vi "Log Write.vi"(0 "Error In":errorcluster, 1 "Write Header":bool, 5 "Log Handle In":T1, 7 "Trajectory In":refnum<data-value>, 9 "State Estimate In":refnum<data-value>, 11 "Measurement In":refnum<data-value>, 12 "Controller Data In":refnum<data-value>, 13 "Balance In":refnum<data-value>) -> (3 "Logged Events":string[](array[string]), 4 "Error Out":errorcluster, 6 "Log Handle Out":T1, 8 "Trajectory Out":refnum<data-value>, 10 "State Estimate Out":refnum<data-value>, 14 "Controller Data Out":refnum<data-value>, 15 "Measurement Out":refnum<data-value>)   [LabVIEW 2021]
uses:
  State Estimator/Measurements.ctl
  IMU/IMU Data.ctl
  Steering Motor Encoder/Steering Motor Encoder Data.ctl
  GNSS/GNSS Data.ctl
  State Estimator/State Estimate.ctl
  Log Handle.ctl
  Controller Data.ctl
  Drive Motor/Drive Motor Data.ctl
  Steering Motor/Steering Motor Data.ctl
  Trajectory Control/Trajectory_Control.ctl
panel:
  out "velocity":dbl
  out "GNSS Data.Speed (m/s)":dbl
  out "rollReference":dbl
  out "Balance Out":refnum<data-value>
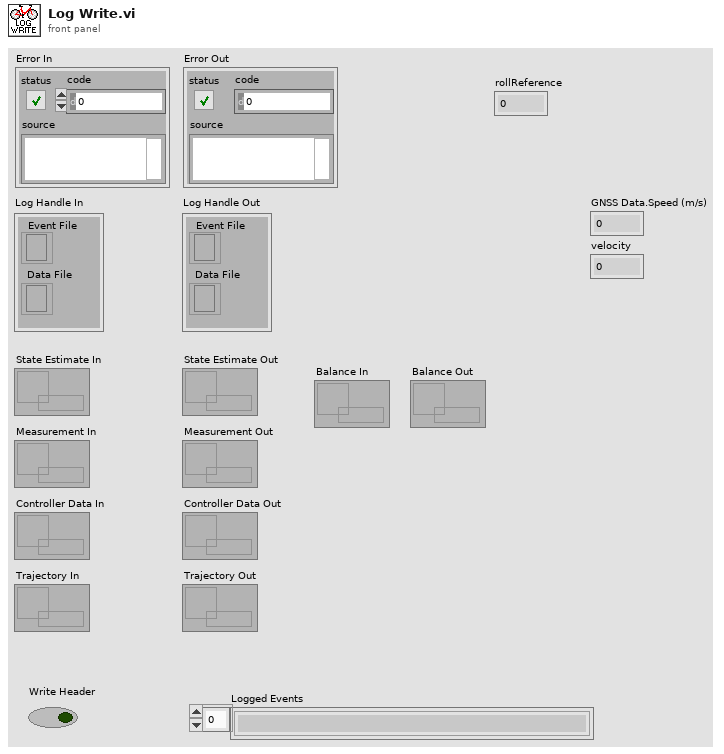
[diagram p1: front panel]
types:
  T1 = typedef "Log Handle.ctl" = cluster{"Data File":refnum<file>, "Event File":refnum<file>}
  T2 = typedef "Controller Data.ctl" = cluster{"Drive Motor Data":T3, "Steering Motor Data":T4}
  T3 = typedef "Drive Motor Data.ctl" = cluster{"Angular Speed (rad/s)":dbl, "Input Current (A)":dbl, "Motor Current (A)":dbl, "MOSFET Temperature (deg C)":dbl, "Reference Speed (rad/s)":dbl, "PI Current (A)":dbl, "Ki":dbl, "Kp":dbl}
  T4 = typedef "Steering Motor Data.ctl" = cluster{"PWM":dbl, "Steering Angle Rate (rad/s)":dbl, "input balancing":dbl}
  T5 = typedef "Trajectory_Control.ctl" = cluster{"Rollref":dbl, "Closestpoint":dbl, "Error1":dbl, "Error2":dbl, "Dpsiref_cont":dbl, "Lateral_cont":dbl, "Heading_cont":dbl, "Reset_traj":dbl, "Iteration":dbl, "E1 limit":u32, "E2 limit":u32}
  T6 = typedef "State Estimate.ctl" = cluster{"X (m)":dbl, "Y (m)":dbl, "Psi (rad)":dbl, "Roll (rad)":dbl, "Roll Rate (rad/s)":dbl, "delta":dbl, "velocity":dbl, "Iterations":dbl}
  T7 = cluster{"Steering Angle Rate":dbl, "rollReference":dbl, "roll":dbl, "rollRate":dbl, "Kp":dbl, "Kd":dbl, "steering_flag":i32}
  T8 = typedef "Measurements.ctl" = cluster{"IMU Data":T9, "Steering Motor Encoder Data":T10, "GNSS Data":T11}
  T9 = typedef "IMU Data.ctl" = cluster{"Gyroscope":cluster{"X (rad/s)":dbl, "Y (rad/s)":dbl, "Z (rad/s)":dbl}, "Accelerometer":cluster{"X (m/s^2)":dbl, "Y (m/s^2)":dbl, "Z (m/s^2)":dbl}, "Flag IMU":dbl}
  T10 = typedef "Steering Motor Encoder Data.ctl" = cluster{"Encoder Position (counts)":i32, "Steering Angle (rad)":dbl, "Steering Encoder Iteration":dbl}
  T11 = typedef "GNSS Data.ctl" = cluster{"Latitude (rad)":dbl, "Longitude (rad)":dbl, "Altitude (m)":dbl, "Speed (m/s)":dbl, "Heading (rad)":dbl, "Fix Quality":i32, "Number of Satellites":i32, "Latitude (deg)":dbl, "Longitude (deg)":dbl, "Flag GNSS":dbl}
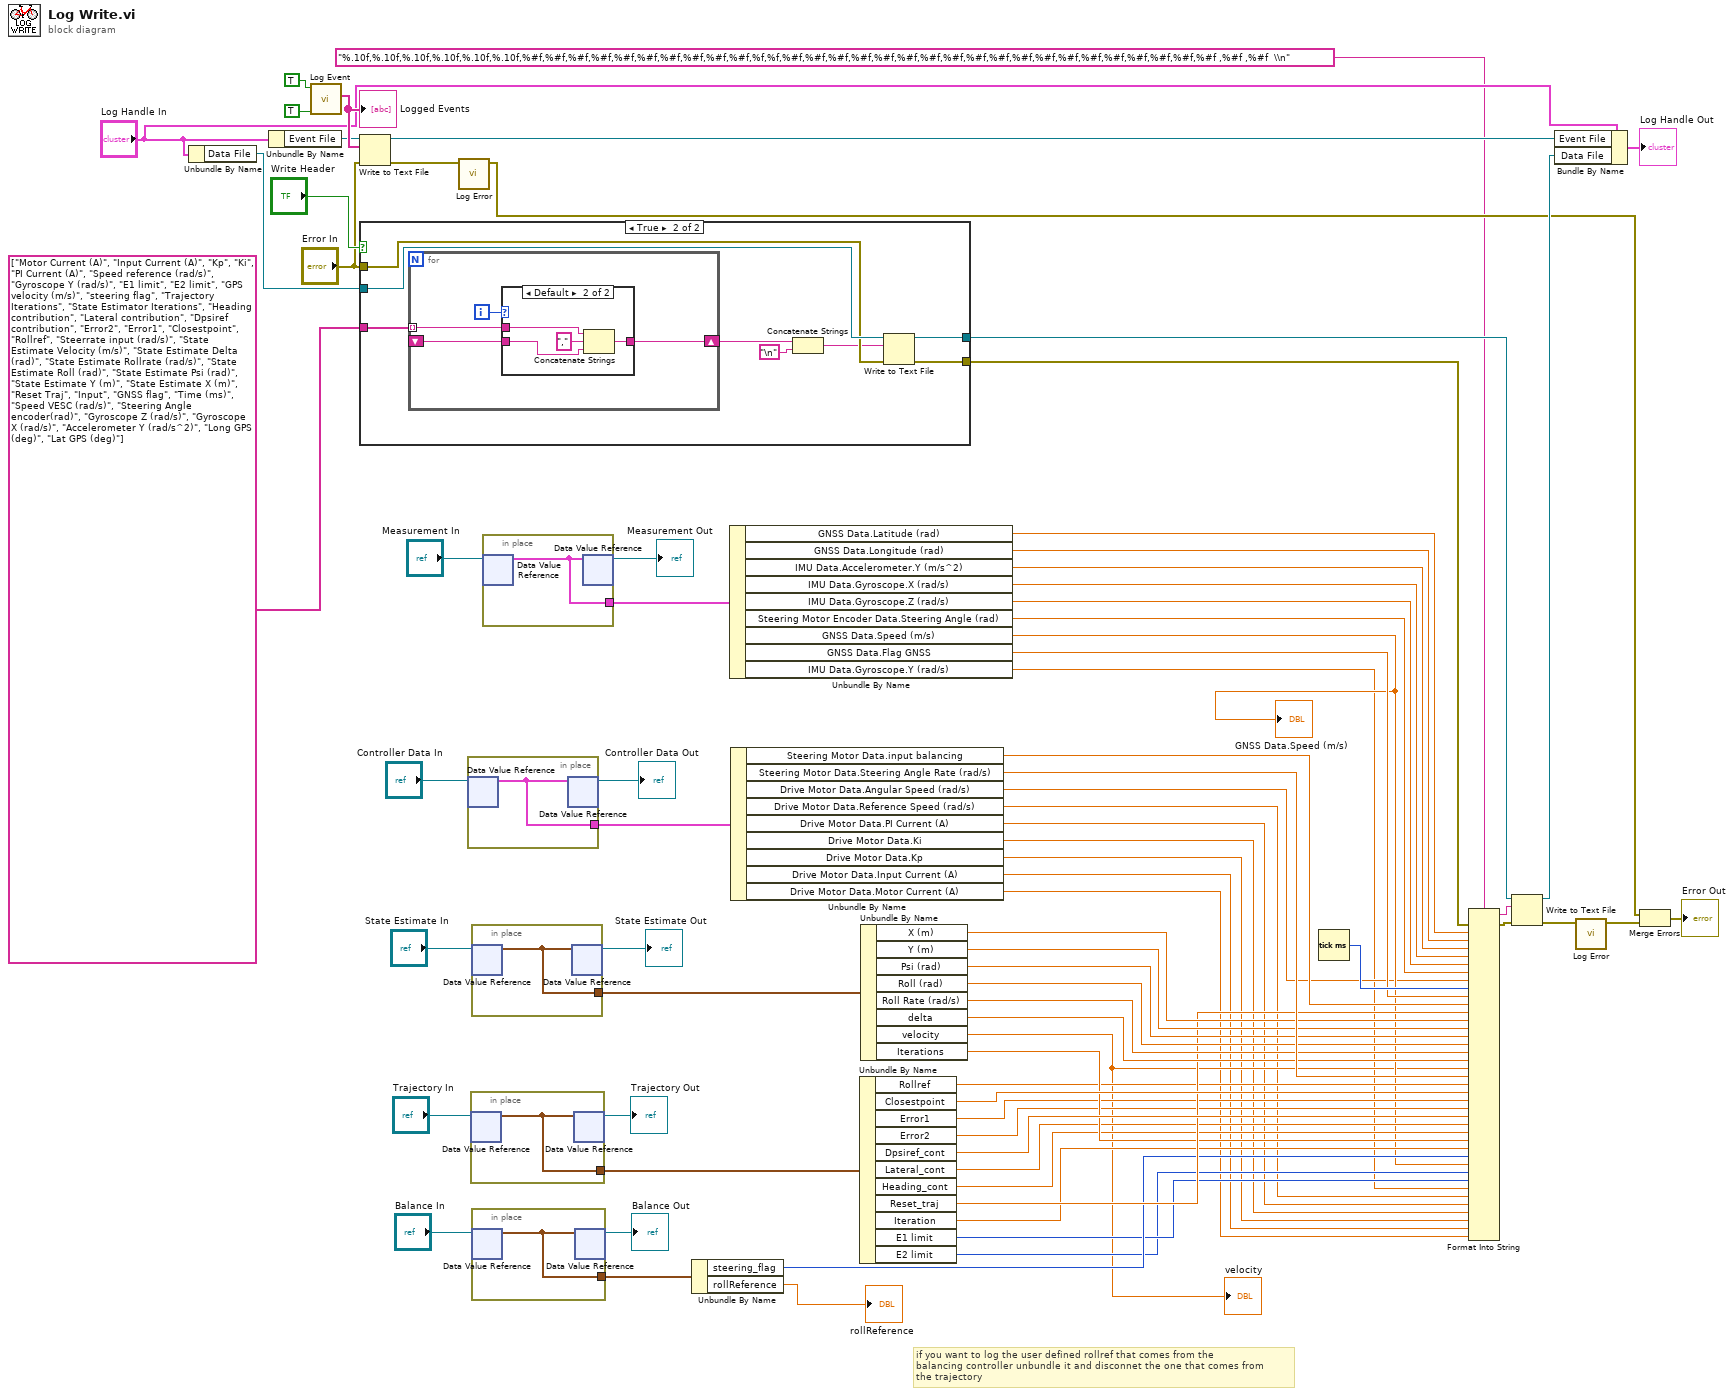
[diagram p0: block diagram]
diagram:
  # "if you want to log the user defined rollref that comes from the \nbalancing controller unbundle it and disconnet the one that comes from \nthe trajectory"
  n1 = Unbundle By Name("Log Handle In") -> ("Data File"=w76:refnum<file>)
  n2 = Unbundle By Name("Log Handle In") -> ("Event File"=w68:refnum<file>)
  n3 = call "Log Event.vi"("Clear Log"=TRUE, "Read"=TRUE) -> ("All Events"=w70:string[])  [unwired: 9 in]
  "Logged Events" <- w70
  n4 = Write to Text File(file (use dialog)=w68, text=w70, error in="Error In") -> (refnum out=w65:refnum<file>, error out=w64:errorcluster)  [unwired: 1 in, 1 out]
  n5 = case shown="True" "Write Header" {
    tunnel: string[] ["Motor Current (A)", "Input Current (A)", "Kp", "Ki", "PI Current (A)", "Speed reference (rad/s)", "Gyroscope Y (rad/s)", "E1 limit", "E2 limit", "GPS velocity (m/s)", "steering flag", "Trajectory Iterations", "State Estimator Iterations", "Heading contribution", "Lateral contribution", "Dpsiref contribution", "Error2", "Error1", "Closestpoint", "Rollref", "Steerrate input (rad/s)", "State Estimate Velocity (m/s)", "State Estimate Delta (rad)", "State Estimate Rollrate (rad/s)", "State Estimate Roll (rad)", "State Estimate Psi (rad)", "State Estimate Y (m)", "State Estimate X (m)", "Reset Traj", "Input", "GNSS flag", "Time (ms)", "Speed VESC (rad/s)", "Steering Angle encoder(rad)", "Gyroscope Z (rad/s)", "Gyroscope X (rad/s)", "Accelerometer Y (rad/s^2)", "Long GPS (deg)", "Lat GPS (deg)"] ("channel name(s) in (Untitled)") -> [_ w87]
    tunnel: w76 -> [w79 w86]
    tunnel: "Error In" -> [w78 w85]
    tunnel: [w79 w84] -> w74
    tunnel: [w78 w83] -> w73
    frame False {
    }
    frame True {
      n6 = for {
        tunnel: w87 -> [w91] mode=indexing
        shift-right: [w89] -> w82
        shift-left: _ -> [w88]
        i -> [w90]
        n7 = case shown="Default" w90 {
          tunnel: w91 -> [w92 w96]
          tunnel: [w92 w95] -> w89
          tunnel: w88 -> [_ w94]
          frame 0 {
          }
          frame Default {
            n8 = Concatenate Strings(w96, "," ("string"), w94) -> (w95:string)
          }
        }
      }
      n9 = Concatenate Strings(w82, "\n") -> (w81:string)
      n10 = Write to Text File(file (use dialog)=w86, text=w81, error in=w85) -> (refnum out=w84:refnum<file>, error out=w83:errorcluster)  [unwired: 1 in, 1 out]
    }
  }
  n11 = call "Log Error.vi"("Error In"=w64) -> ("Error Out"=w62:errorcluster)  [unwired: 10 in]
  n12 = in-place {
    in-place-border: [w97] -> w43
    n13 = in-place-dvr #1("Controller Data In") -> (w97:T2)  [unwired: 1 out]
    n14 = in-place-dvr #1(w97) -> (→"Controller Data Out":refnum<data-value>)  [unwired: 1 out]
  }
  n15 = in-place {
    in-place-border: [w98] -> w31
    n16 = in-place-dvr #2("Trajectory In") -> (w98:T5)  [unwired: 1 out]
    n17 = in-place-dvr #2(w98) -> (→"Trajectory Out":refnum<data-value>)  [unwired: 1 out]
  }
  n18 = in-place {
    in-place-border: [w99] -> w54
    n19 = in-place-dvr #3("State Estimate In") -> (w99:T6)  [unwired: 1 out]
    n20 = in-place-dvr #3(w99) -> (→"State Estimate Out":refnum<data-value>)  [unwired: 1 out]
  }
  n21 = in-place {
    in-place-border: [w100] -> w17
    n22 = in-place-dvr #4("Balance In") -> (w100:T7)  [unwired: 1 out]
    n23 = in-place-dvr #4(w100) -> (→"Balance Out":refnum<data-value>)  [unwired: 1 out]
  }
  n24 = in-place {
    in-place-border: [w101] -> w55
    n25 = in-place-dvr #5("Measurement In") -> (w101:T8)  [unwired: 1 out]
    n26 = in-place-dvr #5(w101) -> (→"Measurement Out":refnum<data-value>)  [unwired: 1 out]
  }
  n27 = Unbundle By Name(w17) -> ("steering_flag"=w16:i32, "rollReference"=→"rollReference":dbl)
  n28 = Unbundle By Name(w55) -> ("GNSS Data.Latitude (rad)"=w34:dbl, "GNSS Data.Longitude (rad)"=w53:dbl, "IMU Data.Accelerometer.Y (m/s^2)"=w52:dbl, "IMU Data.Gyroscope.X (rad/s)"=w51:dbl, "IMU Data.Gyroscope.Z (rad/s)"=w50:dbl, "Steering Motor Encoder Data.Steering Angle (rad)"=w49:dbl, "GNSS Data.Speed (m/s)"=w11:dbl, "GNSS Data.Flag GNSS"=w29:dbl, "IMU Data.Gyroscope.Y (rad/s)"=w8:dbl)
  "GNSS Data.Speed (m/s)" <- w11
  n29 = Unbundle By Name(w43) -> ("Steering Motor Data.input balancing"=w26:dbl, "Steering Motor Data.Steering Angle Rate (rad/s)"=w42:dbl, "Drive Motor Data.Angular Speed (rad/s)"=w10:dbl, "Drive Motor Data.Reference Speed (rad/s)"=w7:dbl, "Drive Motor Data.PI Current (A)"=w6:dbl, "Drive Motor Data.Ki"=w5:dbl, "Drive Motor Data.Kp"=w4:dbl, "Drive Motor Data.Input Current (A)"=w2:dbl, "Drive Motor Data.Motor Current (A)"=w1:dbl)
  n30 = Unbundle By Name(w31) -> ("Rollref"=w14:dbl, "Closestpoint"=w30:dbl, "Error1"=w21:dbl, "Error2"=w20:dbl, "Dpsiref_cont"=w28:dbl, "Lateral_cont"=w23:dbl, "Heading_cont"=w22:dbl, "Reset_traj"=w27:dbl, "Iteration"=w24:dbl, "E1 limit"=w13:u32, "E2 limit"=w12:u32)
  n31 = Unbundle By Name(w54) -> ("X (m)"=w40:dbl, "Y (m)"=w39:dbl, "Psi (rad)"=w38:dbl, "Roll (rad)"=w37:dbl, "Roll Rate (rad/s)"=w36:dbl, "delta"=w35:dbl, "velocity"=w9:dbl, "Iterations"=w25:dbl)
  "velocity" <- w9
  n32 = Tick Count (ms)() -> (millisecond timer value=w41:u32)
  n33 = Format Into String(format string="%.10f,%.10f,%.10f,%.10f,%.10f,%.10f,%#f,%#f,%#f,%#f,%#f,%#f,%#f,%#f,%#f,%#f,%f,%f,%#f,%#f,%#f,%#f,%#f,%#f,%#f,%#f,%#f,%#f,%#f,%#f,%#f,%#f,%#f,%#f,%#f,%#f,%#f ,%#f ,%#f  \\n", error in=w73, w34, w53, w52, w51, w50, w49, w10, w41, w29, w26, w27, w40, w39, w38, w37, w36, w35, w9, w42, w14, w30, w21, w20, w28, w23, w22, w25, w24, w16, w11, w12, w13, w8, w7, w6, w5, w4, w2, w1) -> (resulting string=w48:string, error out=w47:errorcluster)  [unwired: 1 in]
  n34 = Write to Text File(file (use dialog)=w74, text=w48, error in=w47) -> (refnum out=w66:refnum<file>, error out=w46:errorcluster)  [unwired: 1 in, 1 out]
  n35 = Bundle By Name(cluster="Log Handle In", "Event File"=w65, "Data File"=w66) -> (→"Log Handle Out":T1)
  n36 = call "Log Error.vi"("Error In"=w46) -> ("Error Out"=w63:errorcluster)  [unwired: 10 in]
  n37 = Merge Errors(w62, w63) -> (→"Error Out":errorcluster)
